vi "FTW-JSON-Object-GetElements-String.vi"(0 "JSON Object":refnum<class "FTW-JSON.lvclass">, 5 "Keys":string[](array[string]), 11 "error in":errorcluster) -> (4 "JSON Object out":refnum<class "FTW-JSON.lvclass">, 6 "Values":string[](array[string]), 8 "All Found?":bool, 10 "Which Found?":bool[](array[boolean]), 15 "error out":errorcluster)   [LabVIEW 2013, in "FTW-JSON.lvclass"]
uses:
  FTW-JSON.lvclass
  FTW-JSON.lvclass/FTW-JSON.ctl
panel:
  # "Inputs"
  # "Outputs"
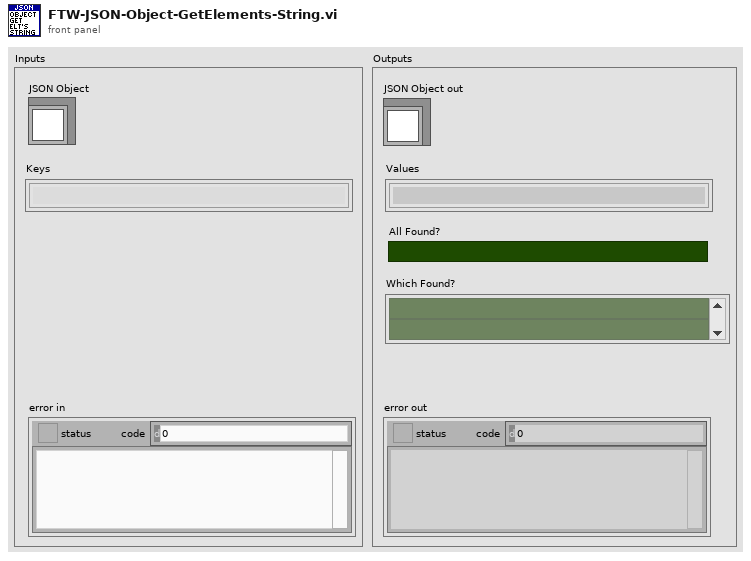
[diagram p1: front panel]
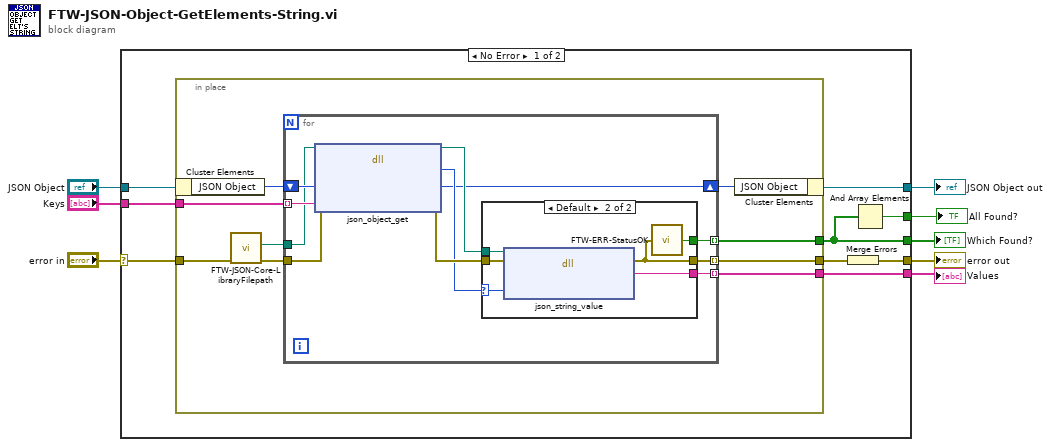
[diagram p0: block diagram]
diagram:
  n1 = case shown="No Error" "error in" {
    selector: "error in" -> [w17 w46]
    tunnel: [w11 w46] -> w8
    tunnel: [w15 w45] -> w6
    tunnel: "JSON Object" -> [w16 w45]
    tunnel: "Keys" -> [w14 _]
    tunnel: [w12 _] -> w1
    tunnel: [w10 _] -> w3
    tunnel: [w9 _] -> w2
    frame No Error {
      n2 = in-place {
        in-place-border: w17 -> [w26]
        in-place-border: w14 -> [w24]
        in-place-border: [w21] -> w13
        in-place-border: [w20] -> w12
        in-place-border: [w18] -> w10
        n3 = in-place-cluster #1(w16) -> ("JSON Object"=w25:i64)
        n4 = call "FTW-JSON-Core-LibraryFilepath.vi"("error in"=w26) -> ("error out"=w23:errorcluster, "JSON Library Filepath"=w22:path)  [unwired: 9 in]
        n5 = for {
          tunnel: w24 -> [w36] mode=indexing
          tunnel: w23 -> [w35]
          tunnel: w22 -> [w34]
          tunnel: [w32] -> w21 mode=indexing
          tunnel: [w31] -> w20 mode=indexing
          tunnel: [w27] -> w18 mode=indexing
          shift-right: [w28] -> w19
          shift-left: w25 -> [w37]
          n6 = dll-call lib="?" fn="json_object_get"(path in=w34, error in=w35, "JSON Object Pointer"=w37, "Element Key"=w36) -> (path out=w30:path, error out=w33:errorcluster, "JSON Element Pointer"=w29:i64, "JSON Object Pointer"=w28:i64)  [unwired: 2 in]
          n7 = case shown="Default" w29 {
            selector: w29 -> [_ w41]
            tunnel: w33 -> [w38 w44]
            tunnel: [w38 w40] -> w32
            tunnel: [_ w43] -> w31
            tunnel: w30 -> [_ w42]
            tunnel: [_ w39] -> w27
            frame 0 {
            }
            frame Default {
              n8 = dll-call lib="?" fn="json_string_value"(path in=w42, error in=w44, "JSON Element Pointer"=w41) -> (error out=w40:errorcluster, "String Value"=w43:string)  [unwired: 2 in, 1 out]
              n9 = call "FTW-ERR-StatusOK.vi"("error to check"=w40) -> ("Status OK?"=w39:bool)
            }
          }
        }
        n10 = in-place-cluster #1("JSON Object"=w19) -> (w15:refnum<class "FTW-JSON.lvclass">)
      }
      n11 = Merge Errors(w13) -> (w11:errorcluster)
      n12 = And Array Elements(Boolean array=w10) -> (logical AND=w9:bool)
    }
    frame Error {
    }
  }
  "error out" <- w8
  "JSON Object out" <- w6
  "Which Found?" <- w3
  "All Found?" <- w2
  "Values" <- w1
